vi "Command.vi"(8 "error in (no error)":errorcluster, 9 "Microscope events":T1, 10 "Stage events":T2, 11 "Microscope in":refnum<class "Microscope.lvclass">) -> (0 "error out":errorcluster, 3 "Microscope out":refnum<class "Microscope.lvclass">)   [LabVIEW 2012, in "Microscope.lvclass"]
uses:
  classes/Microscope.lvclass
  typedefs/StageEvent.ctl
  typedefs/MicroscopeEvent.ctl
  classes/Microscope.lvclass/Microscope.ctl
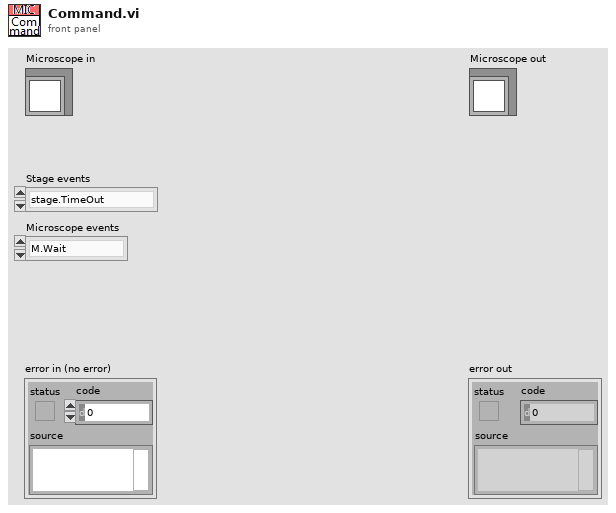
[diagram p1: front panel]
types:
  T1 = typedef "MicroscopeEvent.ctl" = enum16{"M.Wait", "M.RunRotation", "M.Flush", "M.Init", "M.InitStage", "M.InitImageData", "M.ReinitImageData", "M.ReinitImageParams", "M.GetSetParams", "M.InitFastHardware", "M.Pre-Acquire", "M.Acquire", "M.PostAcquire", "M.StopAcquire", "M.SetAcqStatusTrue", "M.SetAcqStatusFalse", "M.ClearImageData", "M.MoveStageDiscrete", "M.MoveStageToTarget1", "M.MoveStageToTarget2", "M.MoveStageToTarget3", "M.OpenShutters", "M.CloseShutters", "M.StartAcquireSequence", "M.ChangeParameters", "M.OpenStokes", "M.OpenPump", "M.RunSW"}
  T2 = typedef "StageEvent.ctl" = enum16{"stage.TimeOut", "stage.FlushData", "stage.GetPosition", "stage.Init", "stage.MoveTo1", "stage.MoveTo2", "stage.MoveTo3", "stage.Stop"}
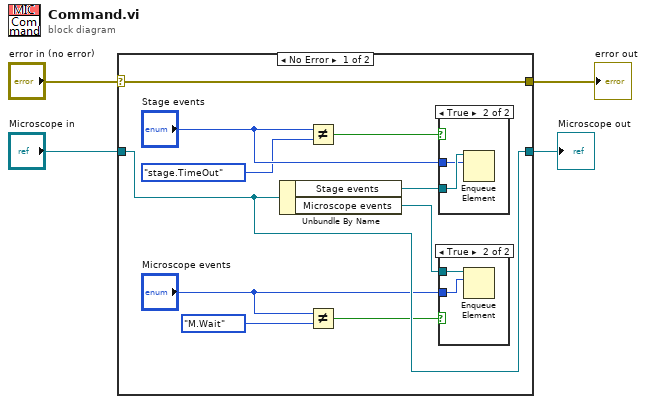
[diagram p0: block diagram]
diagram:
  n1 = case shown="No Error" "error in (no error)" {
    selector: "error in (no error)" -> [w14 w20]
    tunnel: [w14 w20] -> w3
    tunnel: [w13 w19] -> w1
    tunnel: "Microscope in" -> [w13 w19]
    frame No Error {
      n2 = Unbundle By Name(w13) -> ("Stage events"=w12:refnum<queue>, "Microscope events"=w6:refnum<queue>)
      n3 = Not Equal?(x="Stage events", y=StageEvent."stage.TimeOut") -> (x != y?=w9:bool)
      n4 = Not Equal?(x="Microscope events", y=MicroscopeEvent."M.Wait") -> (x != y?=w7:bool)
      n5 = case shown="True" w9 {
        tunnel: w12 -> [_ w18]
        tunnel: "Stage events" -> [_ w17]
        frame False {
        }
        frame True {
          n6 = Enqueue Element(queue=w18, element=w17) -> ()  [unwired: 2 in, 3 out]
        }
      }
      n7 = case shown="True" w7 {
        tunnel: w6 -> [_ w16]
        tunnel: "Microscope events" -> [_ w15]
        frame False {
        }
        frame True {
          n8 = Enqueue Element(queue=w16, element=w15) -> ()  [unwired: 2 in, 3 out]
        }
      }
    }
    frame Error {
    }
  }
  "error out" <- w3
  "Microscope out" <- w1
